vi "Hough's Transform.vi"(3 "Error":string, 4 "Hough's Transform's Result":i16, 5 "Input Image":T1={"Image ID"=0, "Channel ID"=-1}) -> (0 "Error":string, 1 "Hough's Transform's Result":i16, 2 "Input Image":T1={"Image ID"=0, "Channel ID"=-1})   [LabVIEW 2011, in "labvvis.lvlib"]
doc: "Returns an array with 256 elements, where each element in the array contains the number of times pixels equal to the index is encountered in Input Image.\n\nIf you connect an array that does not have 256 elements, this VI will not execute. If you do not connect an array at all, this VI will provide one.\n\nNote that this VI only operates on single-channel images. Thus grey-scale, Red channel, Green channel and so on images are supported. RGBA images are not supported."
uses:
  <userlib>/labvvis/labvvis.lvlib
  <userlib>/labvvis/VVIS Image.ctl
  labvvis.framework
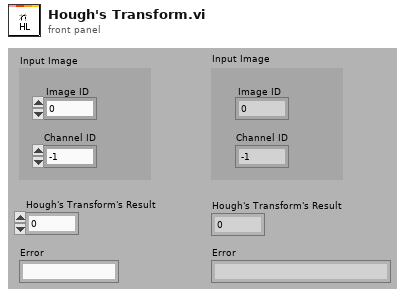
[diagram p1: front panel]
types:
  T1 = typedef "labvvis.lvlib/VVIS Image.ctl" = cluster{"Image ID":i16, "Channel ID":i16}
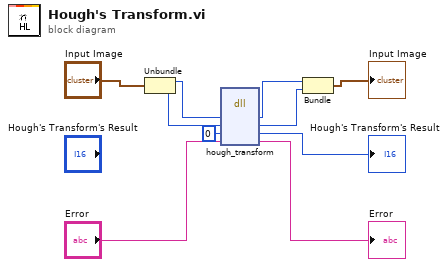
[diagram p0: block diagram]
diagram:
  n1 = Unbundle("Input Image") -> ("Image ID"=w9:i16, "Channel ID"=w8:i16)
  n2 = dll-call lib="labvvis.framework" fn="hough_transform"("src1"=w9, "cid"=w8, "hough_id"=i16 0, "error"="Error") -> ("src1"=w7:i16, "cid"=w6:i16, "hough_id"=→"Hough's Transform's Result":i16, "error"=→"Error":string)  [unwired: 4 in, 2 out]
  n3 = Bundle("src1"=w7, "cid"=w6) -> (→"Input Image":cluster{"src1":i16, "cid":i16})  [unwired: 1 in]
